vi "PYTHON Get Complex Matrix.vi"(4 "error in (no error)":errorcluster, 5 "data type":cdb[][](array[numeric]) format="%.2f", 6 "variable name":string, 7 "Python Session in":T1) -> (0 "error out":errorcluster, 1 "value":cdb[][](array[numeric]) format="%.2f", 3 "Python Session out":T1)   [LabVIEW 2009]
uses:
  PYTHON Session Refnum.ctl
  lvpython.dll
panel:
  # "PYTHON Get Complex Matrix.vi\n\nGet the value of a complex matrix variable from the session context\n\nCopyright (C) 2002 Rolf Kalbermatter rolf.kalbermatter@citeng.com\nCopyright (C) 2002 James Kring jim@jimkring.com\n\nPlease visit http://www.OpenG.org to learn about the\nOpen Source LabVIEW software movement.\n\nThis library is free software; you can redistribute it and/or\nmodify it under the terms of the GNU Lesser General Public\nLicense as published by the Free Software Foundation; either\nversion 2.1 of the License, or (at your option) any later version.\nThis library is distributed in the hope that it will be useful,\nbut WITHOUT ANY WARRANTY; without even the implied warranty of\nMERCHANTABILITY or FITNESS FOR A PARTICULAR PURPOSE. See the GNU\nLesser General Public License for more details.\nYou should have received a copy of the GNU Lesser General Public\nLicense along with this library; if not, write to the Free Software\nFoundation, Inc., 59 Temple Place, Suite 330, Boston, MA 02111-1307 USA"
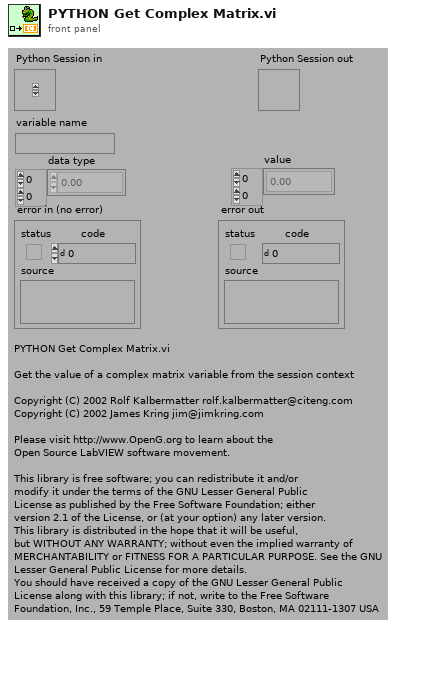
[diagram p1: front panel]
types:
  T1 = typedef "PYTHON Session Refnum.ctl" = refnum<k1>
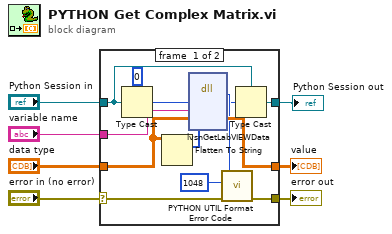
[diagram p0: block diagram]
diagram:
  n1 = case shown="No Error" "error in (no error)" {
    selector: "error in (no error)" -> [w18 w23]
    tunnel: [w8 w22] -> w1
    tunnel: [w17 w23] -> w6
    tunnel: "Python Session in" -> [w9 w22]
    tunnel: "variable name" -> [w20 _]
    tunnel: "data type" -> [w13 w21]
    tunnel: [w19 w21] -> w4
    frame #0 {
      n2 = Type Cast(type=u32 0 ("session"), x=w9) -> (*(type *) &x=w12:u32)
      n3 = Flatten To String(anything=w13) -> (type string=w14:i16[])  [unwired: 3 in, 2 out]
      n4 = dll-call lib="D:/openg/labpython/source/lvpython.*" fn="lvsnGetLabVIEWData"("session"=w12, "name"=w20, "data type"=w13, "type"=w14) -> (w16:i32, "session"=w10:u32, "data type"=w19:cdb[][])  [unwired: 5 in, 2 out]
      n5 = call "PYTHON UTIL Format Error Code.vi"("error in (no error)"=w18, "code"=1048, "Bool32"=w16) -> ("error out"=w17:errorcluster)  [unwired: 4 in]
      n6 = Type Cast(type=w9, x=w10) -> (*(type *) &x=w8:T1)
    }
    frame #1 {
    }
  }
  "error out" <- w6
  "value" <- w4
  "Python Session out" <- w1
